vi "Main_15a.vi"() -> ()   [LabVIEW 2020]
uses:
  Problem-23/Cluster _Point Location.ctl
  Cluster _Point.ctl
panel:
  out "Distances":i32[](array[numeric])
  out "Example 2":string
  out "Beacons":T1[](array[typedef])
  out "Sensors":T1[](array[typedef])
  out "Answer":i32
  in  "Puzzle":string="Sensor at x=1518415, y=2163633: closest beacon is at x=1111304, y=1535696\nSensor at x=2474609, y=3598166: closest beacon is at x=2691247, y=4007257\nSensor at x=426959, y=473371: closest beacon is at x=-529106, y=1145419\nSensor at x=3999598, y=1984775: closest beacon is at x=3975468, y=2000000\nSensor at x=2459256, y=2951561: closest beacon is at x=2132806, y=2866452\nSensor at x=2925882, y=2862933: closest beacon is at x=3325001, y=3024589\nSensor at x=3539174, y=3882566: closest beacon is at x=3132375, y=3541509\nSensor at x=3044887, y=3798155: closest beacon is at x=3132375, y=3541509\nSensor at x=1792818, y=3506985: closest beacon is at x=2132806, y=2866452\nSensor at x=3761945, y=3304667: closest beacon is at x=3325001, y=3024589\nSensor at x=71968, y=3823892: closest beacon is at x=-1085197, y=3401157\nSensor at x=2902345, y=3999748: closest beacon is at x=2691247, y=4007257\nSensor at x=2074989, y=2347435: closest beacon is at x=2132806, y=2866452\nSensor at x=1115220, y=1782338: closest beacon is at x=1111304, y=1535696\nSensor at x=369130, y=2348958: closest beacon is at x=1111304, y=1535696\nSensor at x=2525090, y=1917940: closest beacon is at x=2603675, y=2276026\nSensor at x=2861163, y=3386968: closest beacon is at x=3132375, y=3541509\nSensor at x=3995081, y=2010596: closest beacon is at x=3975468, y=2000000\nSensor at x=3038274, y=534921: closest beacon is at x=4354209, y=-17303\nSensor at x=3646366, y=2868267: closest beacon is at x=3325001, y=3024589\nSensor at x=3308360, y=1653497: closest beacon is at x=3975468, y=2000000\nSensor at x=1996072, y=995783: closest beacon is at x=1111304, y=1535696\nSensor at x=3852158, y=950900: closest beacon is at x=3975468, y=2000000\nSensor at x=3061849, y=2428914: closest beacon is at x=2603675, y=2276026\nSensor at x=2788254, y=3983003: closest beacon is at x=2691247, y=4007257\nSensor at x=694411, y=1882565: closest beacon is at x=1111304, y=1535696\nSensor at x=2647250, y=2551966: closest beacon is at x=2603675, y=2276026\nSensor at x=1079431, y=3166226: closest beacon is at x=2132806, y=2866452\nSensor at x=3929172, y=2196495: closest beacon is at x=3975468, y=2000000\nSensor at x=3883296, y=2487406: closest beacon is at x=3975468, y=2000000\nSensor at x=1271911, y=1529880: closest beacon is at x=1111304, y=1535696"
  in  "Example":string="Sensor at x=2, y=18: closest beacon is at x=-2, y=15\nSensor at x=9, y=16: closest beacon is at x=10, y=16\nSensor at x=13, y=2: closest beacon is at x=15, y=3\nSensor at x=12, y=14: closest beacon is at x=10, y=16\nSensor at x=10, y=20: closest beacon is at x=10, y=16\nSensor at x=14, y=17: closest beacon is at x=10, y=16\nSensor at x=8, y=7: closest beacon is at x=2, y=10\nSensor at x=2, y=0: closest beacon is at x=2, y=10\nSensor at x=0, y=11: closest beacon is at x=2, y=10\nSensor at x=20, y=14: closest beacon is at x=25, y=17\nSensor at x=17, y=20: closest beacon is at x=21, y=22\nSensor at x=16, y=7: closest beacon is at x=15, y=3\nSensor at x=14, y=3: closest beacon is at x=15, y=3\nSensor at x=20, y=1: closest beacon is at x=15, y=3"
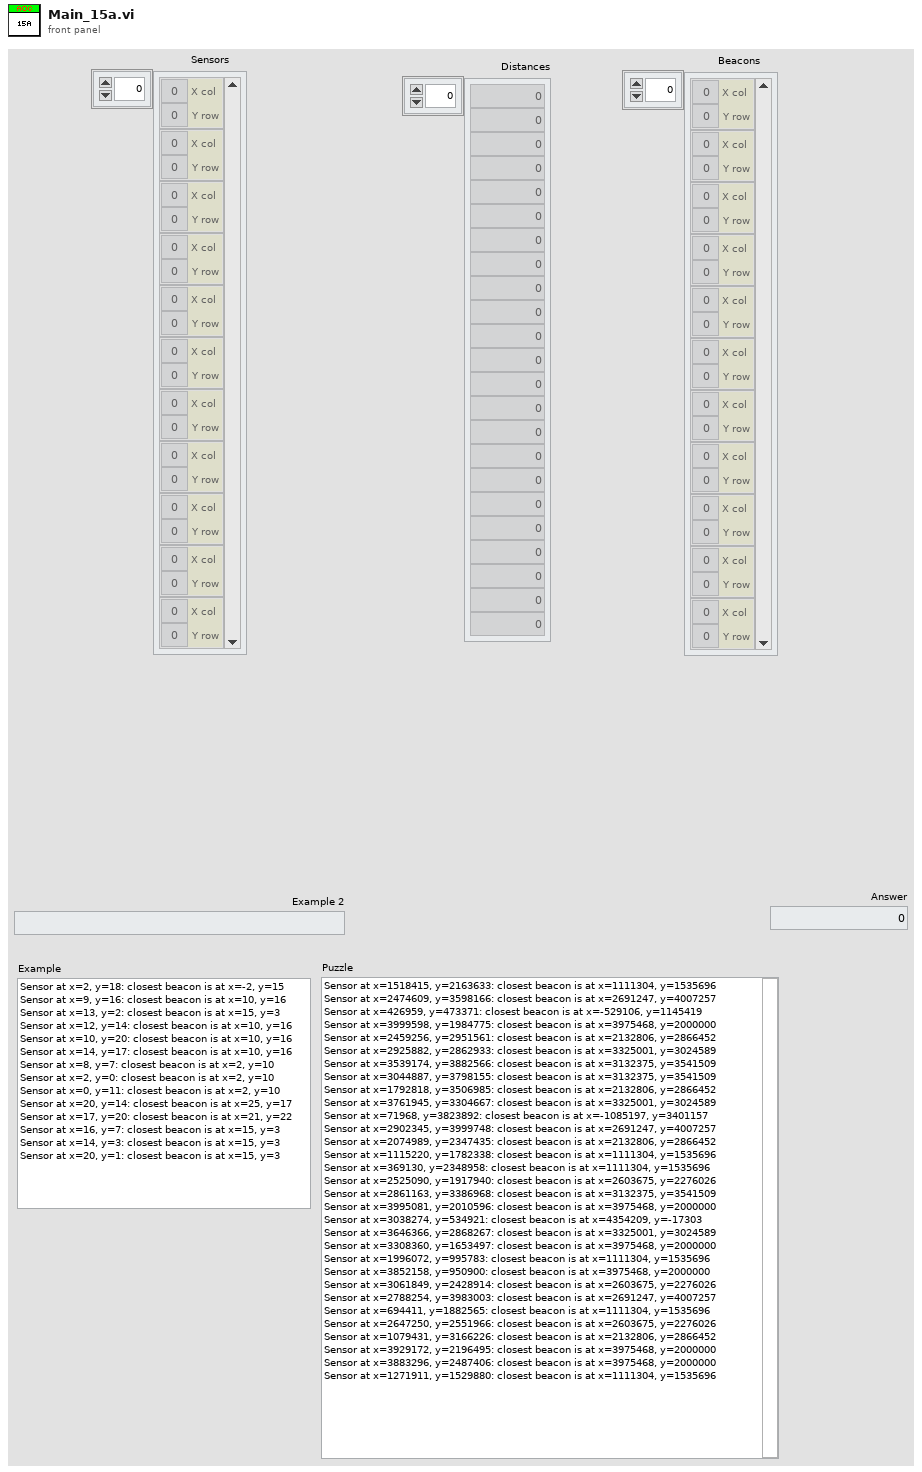
[diagram p1: front panel]
types:
  T1 = typedef "Cluster _Point.ctl" = cluster{"X col":i32, "Y row":i32}
  T2 = typedef "Cluster _Point Location.ctl" = cluster{"X col":i32, "Y row":i32}
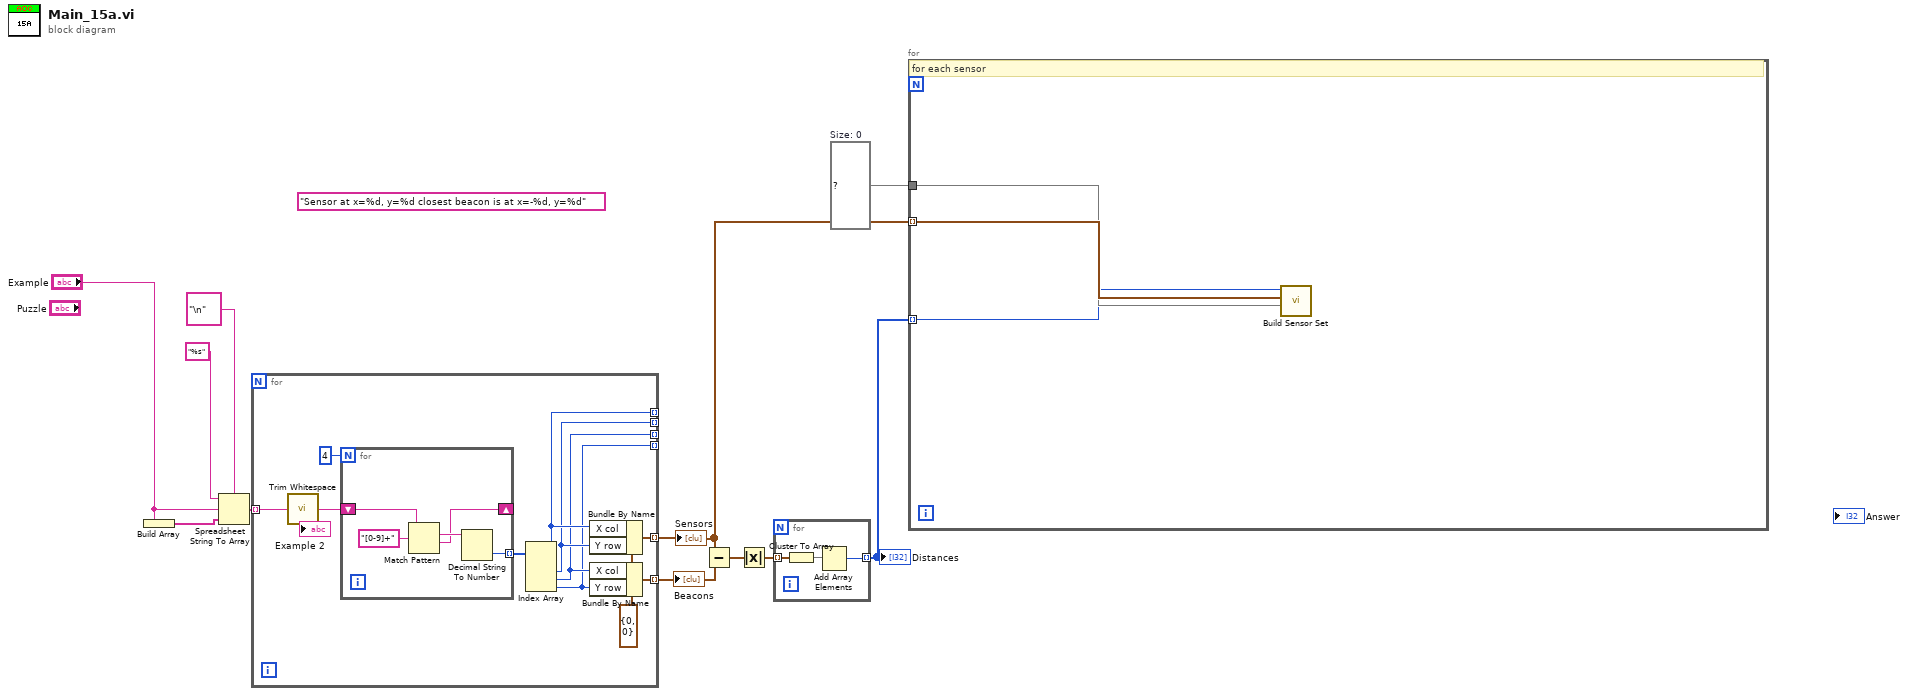
[diagram p0: block diagram]
diagram:
  w1 = set{T2} {}  # Size: 0
  (unwired) "Sensor at x=%d, y=%d closest beacon is at x=-%d, y=%d"
  n1 = Build Array("Example") -> (w11:string[])
  n2 = Spreadsheet String To Array(delimiter (Tab)="\n", format string="%s", spreadsheet string="Example", array type (2D Dbl)=w11) -> (array=w7:string[])
  n3 = for {
    tunnel: w7 -> [w22] mode=indexing
    tunnel: [w21] -> w2 mode=indexing
    tunnel: [w20] -> w6 mode=indexing
    tunnel: [w16] -> _ mode=indexing
    tunnel: [w15] -> _ mode=indexing
    tunnel: [w14] -> _ mode=indexing
    tunnel: [w13] -> _ mode=indexing
    w12 = T1 {"X col"=0, "Y row"=0} ("Point")
    n4 = call <vilib>:"Trim Whitespace.vi"("string"=w22) -> ("trimmed string"=w19:string)  [unwired: 1 in]
    "Example 2" <- w19
    n5 = for {
      N: 4 -> [_]
      shift-right: [w24] -> _
      shift-left: w19 -> [w25]
      tunnel: [w23] -> w17 mode=indexing
      n6 = Match Pattern(string=w25, regular expression="[0-9]+") -> (match substring=w26:string, after substring=w24:string)  [unwired: 1 in, 2 out]
      n7 = Decimal String To Number(string=w26) -> (number=w23:i32)  [unwired: 2 in, 1 out]
    }
    n8 = Index Array(array=w17) -> (element #1=w16:i32, element #2=w15:i32, element #3=w14:i32, element #4=w13:i32)  [unwired: 4 in]
    n9 = Bundle By Name(cluster=w12, "X col"=w16, "Y row"=w15) -> (w21:T1)
    n10 = Bundle By Name(cluster=w12, "X col"=w14, "Y row"=w13) -> (w20:T1)
  }
  "Sensors" <- w2
  "Beacons" <- w6
  n11 = Subtract(x=w2, y=w6) -> (x-y=w5:T1[])
  n12 = Absolute Value(x=w5) -> (abs(x)=w4:T1[])
  n13 = for {
    tunnel: w4 -> [w30] mode=indexing
    tunnel: [w28] -> w3 mode=indexing
    n14 = Cluster To Array(cluster=w30) -> (array=w29:i32[])
    n15 = Add Array Elements(numeric array=w29) -> (sum=w28:i32)
  }
  "Distances" <- w3
  n16 = for {
    tunnel: w3 -> [w31] mode=indexing
    tunnel: w2 -> [w33] mode=indexing
    tunnel: w1 -> [w32]
    # "for each sensor"
    n17 = call "Build Sensor Set.vi"(9:w32, "Distance"=w33, "Point"=w31) -> ()  [unwired: 8 in, 1 out]
  }
